vi "Dispose.vi"(8 "error in (no error)":errorcluster, 11 "CreatorB":refnum<class "CreatorB.lvclass">) -> (0 "error out":errorcluster)   [LabVIEW 2020, in "FactoryMethod.lvlib" / "FactoryMethodLazyEvaluation.lvlib" / "CreatorB.lvclass"]
uses:
  CreatorB.lvclass
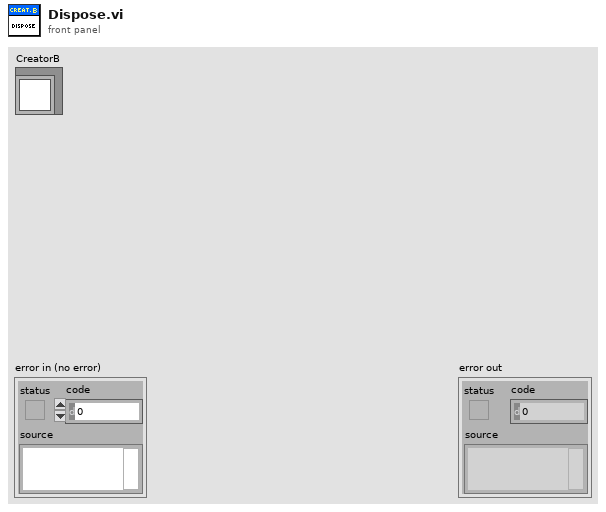
[diagram p1: front panel]
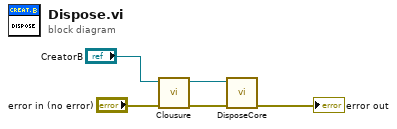
[diagram p0: block diagram]
diagram:
  n1 = call-dynamic "Clousure.vi"("error in (no error)"="error in (no error)", "CreatorB"="CreatorB") -> ("error out"=w3:errorcluster, "CreatorB"=w2:refnum<class "CreatorB.lvclass">)  [unwired: 8 in]
  n2 = call-dynamic "DisposeCore.vi"("error in (no error)"=w3, "CreatorB"=w2) -> ("error out"=→"error out":errorcluster)  [unwired: 8 in, 1 out]
